vi "DBL Variant or Array Variant to Array.vi"(8 "error in (no error)":errorcluster, 11 "value":variant) -> (0 "error out":errorcluster, 3 "Array":dbl[](array[numeric]))   [LabVIEW 2016, in "Control Experiment.lvclass"]
uses:
  Control Experiment.lvclass
  <vilib>/Utility/Data Type/NI_Data Type.lvlib
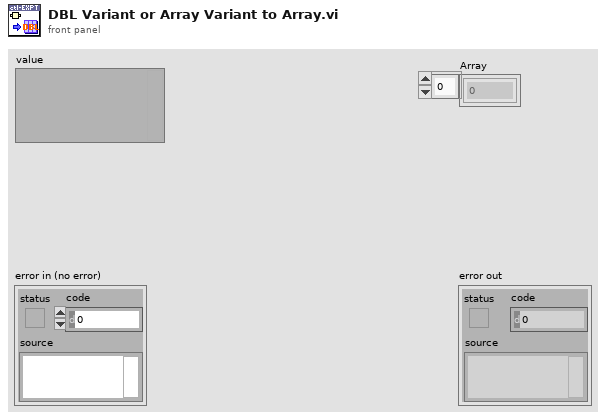
[diagram p1: front panel]
types:
  T1 = typedef "NI_Data Type.lvlib/Data Type.ctl" = enum8{"Invalid Type", "Void", "I8", "I16", "I32", "I64", "U8", "U16", "U32", "U64", "Single Float", "Double Float", "Extended Float", "Single Complex", "Double Complex", "Extended Complex", "Enum U8", "Enum U16", "Enum U32", "Enum U64", "Single Float With Unit", "Double Float With Unit", "Extended Float With Unit", "Single Complex with Unit", "Double Complex with Unit", "Extended Complex with Unit", "Boolean", "String", "Path", "Picture", "Tag", "Array", "Cluster", "Variant", "LV Variant", "Waveform", "Timestamp", "Digital Waveform", "Digital Data", "ExpressData", "Refnum", "External Data", "VI", "Poly VI", "LabVIEW Class Instance", "Fixed Point"}
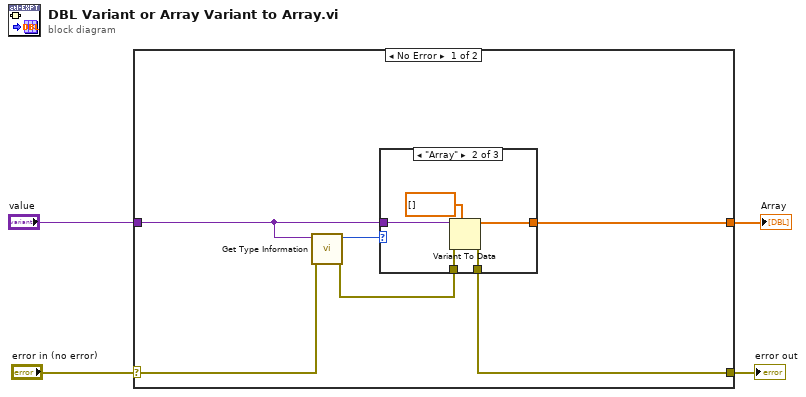
[diagram p0: block diagram]
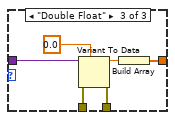
[diagram p3: hidden frame]
diagram:
  n1 = case shown="No Error" "error in (no error)" {
    selector: "error in (no error)" -> [w7 w23]
    tunnel: [w6 w23] -> w3
    tunnel: "value" -> [w9 _]
    tunnel: [w5 _] -> w1
    frame No Error {
      n2 = call <vilib>:"Get Type Information.vi"("error in (no error)"=w7, "Variant"=w9) -> ("error out"=w8:errorcluster, "Type"=w10:T1)  [unwired: 5 in, 3 out]
      n3 = case shown="\"Array\"" w10 {
        tunnel: [w11 w15 w22] -> w6
        tunnel: [_ w14 w17] -> w5
        tunnel: w9 -> [_ w13 w20]
        tunnel: w8 -> [w11 w12 w19]
        frame Default {
        }
        frame "Array" {
          n4 = Variant To Data(error in=w12, type=dbl[] [], Variant=w13) -> (data=w14:dbl[], error out=w15:errorcluster)
        }
        frame "Double Float" {
          n5 = Variant To Data(error in=w19, type=0.0, Variant=w20) -> (data=w21:dbl, error out=w22:errorcluster)
          n6 = Build Array(w21) -> (w17:dbl[])
        }
      }
    }
    frame Error {
    }
  }
  "error out" <- w3
  "Array" <- w1
